vi "Add Item to Tree.vi"(8 "error in (no error)":errorcluster, 10 "Malleable VI Type in":refnum<class "Malleable VI Type.lvclass">, 11 "Tree Ref in":refnum<vi>) -> (0 "error out":errorcluster, 1 "Added Tag":string, 2 "Malleable VI Type out":refnum<class "Malleable VI Type.lvclass">, 3 "Tree Ref out":refnum<vi>)   [LabVIEW 2020, in "Peek Window.lvlib" / "Malleable VI Type.lvclass"]
uses:
  Malleable VI Type.lvclass
  Symbols Enum.ctl
  Malleable VI Type.lvclass/Malleable VI Type.ctl
  Standard VI Type/Standard VI Type.lvclass/Standard VI Type.ctl
  Standard VI Type/Read Full Qualified Name.vi
  Implementation VI Type/Implementation VI Type.lvclass
  D:/Code/VI-Peek/source/Peek Window/VI Types/Standard VI Type/Standard VI Type.lvclass
  Peek Window.lvlib
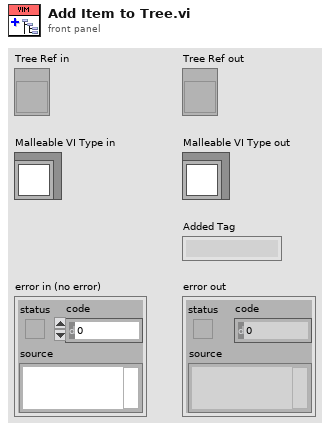
[diagram p1: front panel]
types:
  T1 = typedef "Peek Window.lvlib/Symbols Enum.ctl" = enum16{"<Blank>", "Implementation Mark", "Standard VI", "Dynamic Dispatch VI", "Malleable VI", "Polymorphic VI", "Missing VI", "Express VI"}
  T2 = typedef "Peek Window.lvlib/Malleable VI Type.lvclass/Selected Implementation Enum.ctl" = enum16{"Actual", "Instance"}
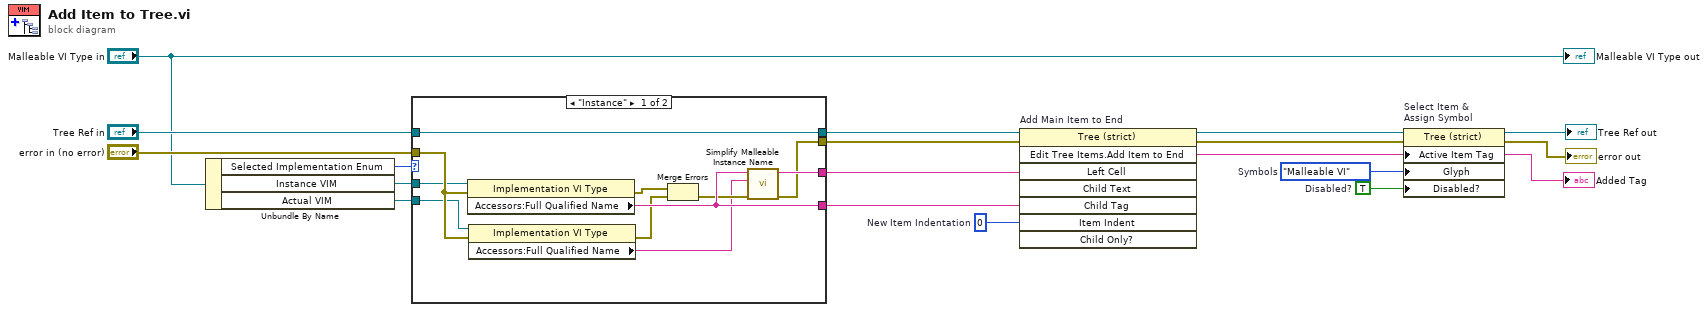
[diagram p0: block diagram]
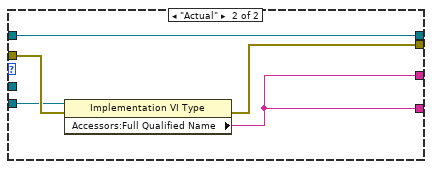
[diagram p2: hidden frame]
diagram:
  w1 = TRUE  # Disabled?
  w15 = Symbols_Enum."Malleable VI"  # Symbols
  w18 = 0  # New Item Indentation
  n1 = Unbundle By Name("Malleable VI Type in") -> ("Selected Implementation Enum"=w5:T2, "Instance VIM"=w3:refnum<class "Implementation VI Type.lvclass">, "Actual VIM"=w2:refnum<class "Implementation VI Type.lvclass">)
  n2 = case shown="\"Instance\"" w5 {
    tunnel: [w29 w31] -> w11
    tunnel: [w28 w31] -> w10
    tunnel: [w27 w32] -> w9
    tunnel: "error in (no error)" -> [w25 w33]
    tunnel: "Tree Ref in" -> [w26 w34]
    tunnel: [w26 w34] -> w6
    tunnel: w3 -> [w21 _]
    tunnel: w2 -> [w20 w30]
    frame "Instance" {
      n3 = property class="Implementation VI Type"(reference=w21, error in=w25) -> (error out=w23:errorcluster, "Accessors:Full Qualified Name"=w29:string)  [unwired: 1 out]
      n4 = property class="Implementation VI Type"(reference=w20, error in=w25) -> (error out=w22:errorcluster, "Accessors:Full Qualified Name"=w19:string)  [unwired: 1 out]
      n5 = Merge Errors(w23, w22) -> (w24:errorcluster)
      n6 = call "Simplify Malleable Instance Name.vi"("error in (no error)"=w24, "Fully Qualified Malleable VI Name"=w19, "Fully Qualified Malleable Instance Name"=w29) -> ("error out"=w27:errorcluster, "Simple Malleable Instance Name"=w28:string)  [unwired: 7 in]
    }
    frame "Actual" {
      n7 = property class="Implementation VI Type"(reference=w30, error in=w33) -> (error out=w32:errorcluster, "Accessors:Full Qualified Name"=w31:string)  [unwired: 1 out]
    }
  }
  n8 = invoke on="Add Main Item to End" class="Tree (strict)" method="Edit Tree Items.Add Item to End"(reference=w6, error in=w9, "Left Cell"=w10, "Child Tag"=w11, "Item Indent"=w18) -> (reference out=w17:refnum<vi>, error out=w16:errorcluster, "Edit Tree Items:Add Item to End"=w12:string)  [unwired: 3 in, 5 out]
  "Added Tag" <- w12
  n9 = property on="Select Item &\nAssign Symbol" class="Tree (strict)"(reference=w17, error in=w16, "Active Item Tag"=w12, "Glyph"=w15, "Disabled?"=w1) -> (reference out=→"Tree Ref out":refnum<vi>, error out=→"error out":errorcluster)
  "Malleable VI Type out" <- "Malleable VI Type in"
